vi "Log Config.vi"(8 "error in (no error)":errorcluster, 11 "Log Config in":T1) -> (0 "error out":errorcluster, 3 "Log Config out":T1={"Log Level"=enum."WARNING"})   [LabVIEW 2020, in "RxnRover.lvlib" / "logging.lvlib"]
doc: "Provides access to read from or write to the log configuration, maintaining a functional global variable of the current configuration state.\n\nWARNING: This VI should not be used to change the logging configuration by itself! It is only intended for internal use. Instead use the Get and Set wrapper functions."
uses:
  logging.lvlib
  Log Levels.ctl
  Log Config.ctl
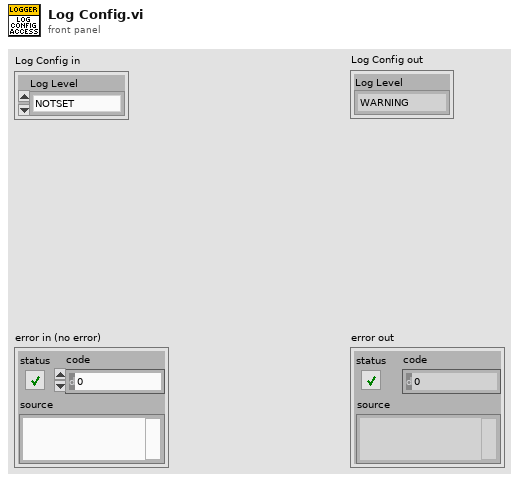
[diagram p1: front panel]
types:
  T1 = typedef "RxnRover.lvlib/logging.lvlib/Log Config.ctl" = cluster{"Log Level":T2}
  T2 = typedef "RxnRover.lvlib/logging.lvlib/Log Levels.ctl" = enum16{"NOTSET", "DEBUG", "INFO", "WARNING", "ERROR", "CRITICAL"}
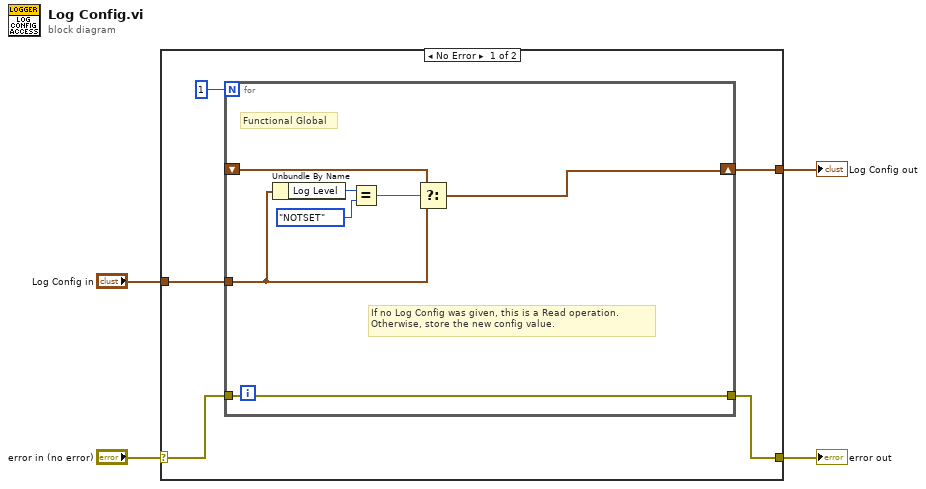
[diagram p0: block diagram]
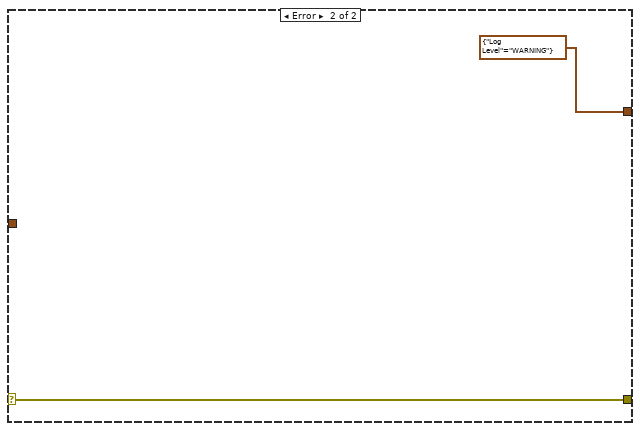
[diagram p2: hidden frame]
diagram:
  n1 = case shown="No Error" "error in (no error)" {
    selector: "error in (no error)" -> [w7 w18]
    tunnel: [w6 w18] -> w3
    tunnel: "Log Config in" -> [w5 _]
    tunnel: [w8 T1 {"Log Level"=enum."WARNING"} ("Log Config out")] -> w1
    frame No Error {
      n2 = for {
        N: 1 -> [_]
        shift-right: [w12] -> w8
        shift-left: _ -> [w10]
        tunnel: w7 -> [w16]
        tunnel: [w16] -> w6
        tunnel: w5 -> [w11]
        # "If no Log Config was given, this is a Read operation. Otherwise, store the new config value."
        # "Functional Global"
        n3 = Unbundle By Name(w11) -> ("Log Level"=w14:T2)
        n4 = Equal?(x=w14, y=Log_Levels."NOTSET" ("Log Level")) -> (x = y?=w13:bool)
        n5 = Select(t=w10, s=w13, f=w11) -> (s? t:f=w12:T1)
      }
    }
    frame Error {
    }
  }
  "error out" <- w3
  "Log Config out" <- w1
